vi "Forbidden.vi"() -> ()   [LabVIEW 2014]
panel:
  in  "menu":bool
  out "forbidden":bool[][](array[boolean])
  out "current col":dbl
  out "current row":dbl
  in  "redo":bool
  out "status":bool
  in  "resume":bool caption="restart"
  out "Game status":string
  out "?":bool
  out "?":bool
  out "counts":dbl
  out "white":bool[][](array[boolean])
  out "blackPiece":bool
  out "whitePiece":bool
  out "black":bool[][](array[boolean])
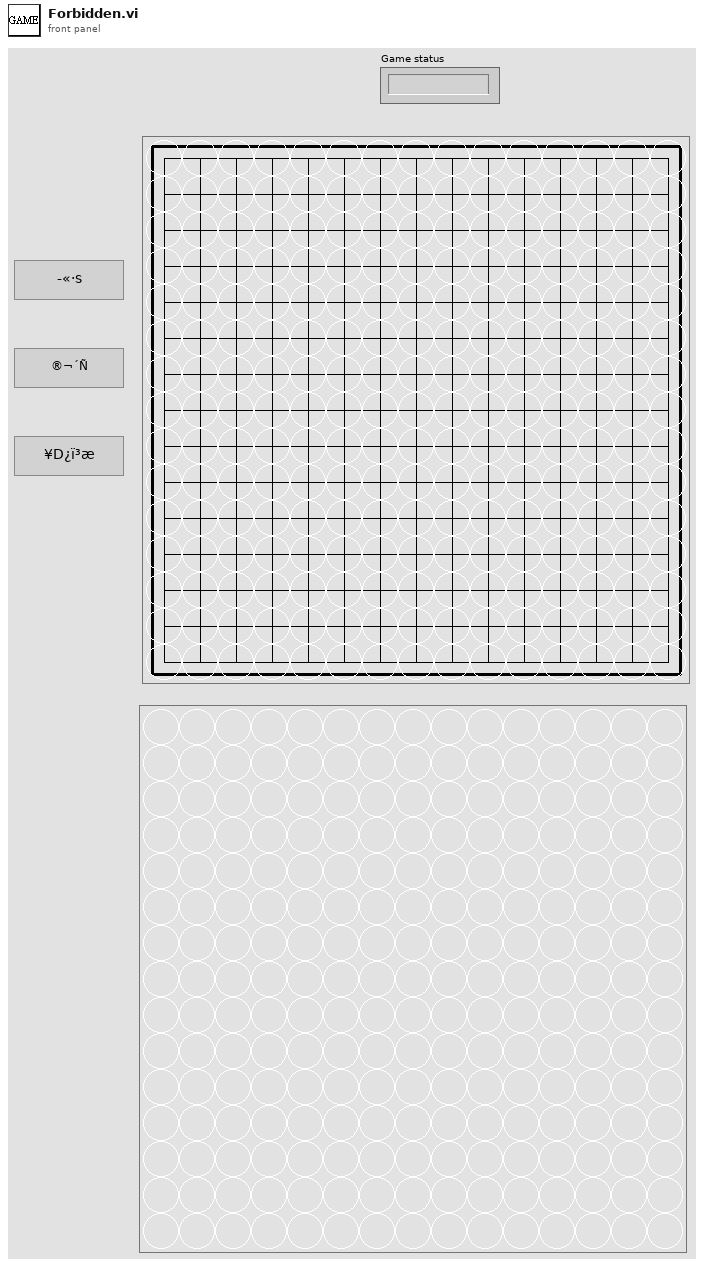
[diagram p1: front panel]
types:
  T1 = typedef "LVPoint32TypeDef.ctl" = cluster{"Horizontal":i32, "Vertical":i32}
  T2 = cluster{"Numeric Control":dbl, "Numeric Control":dbl}
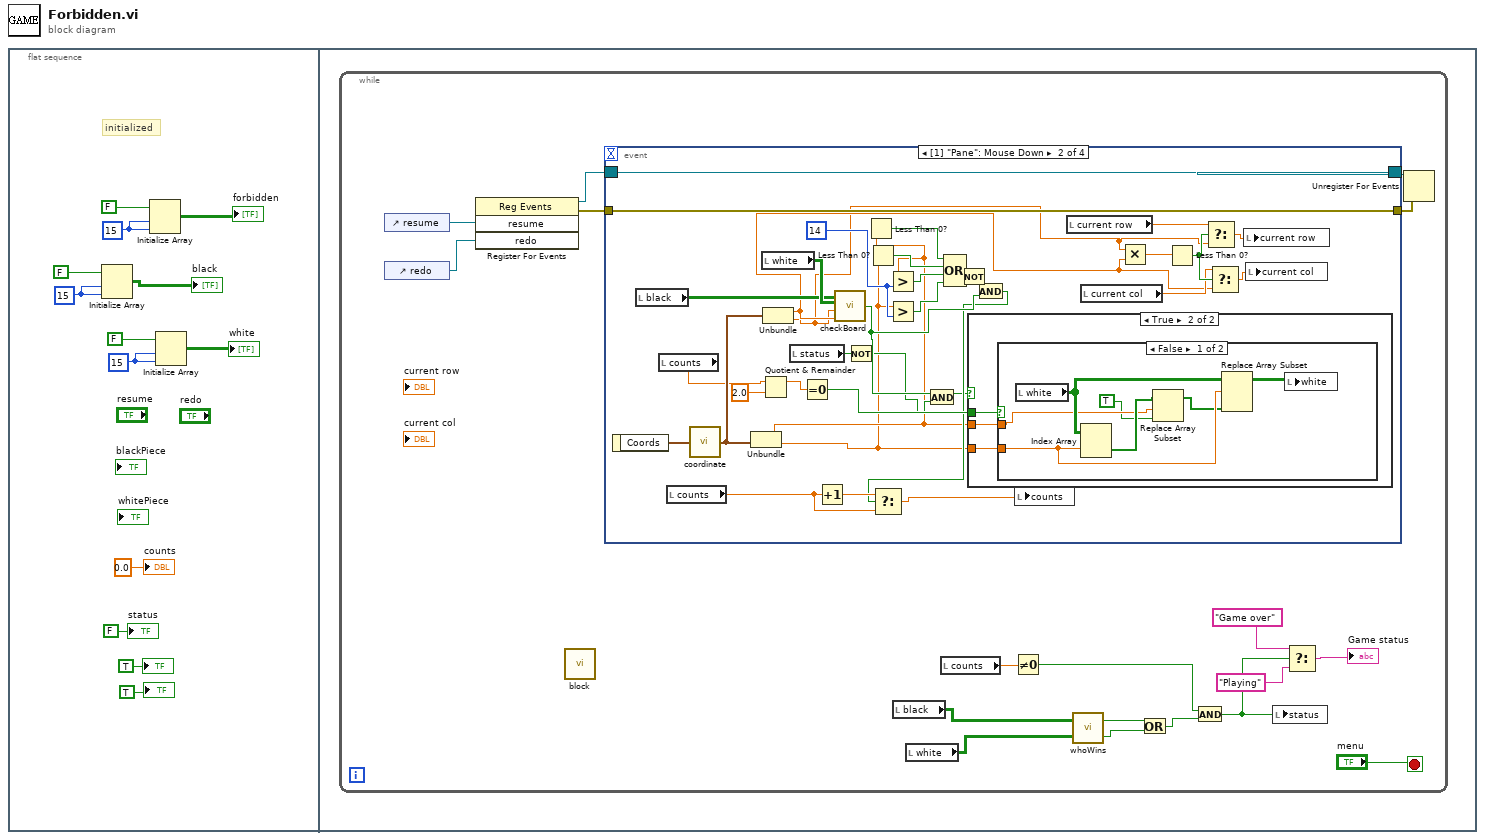
[diagram p0: block diagram]
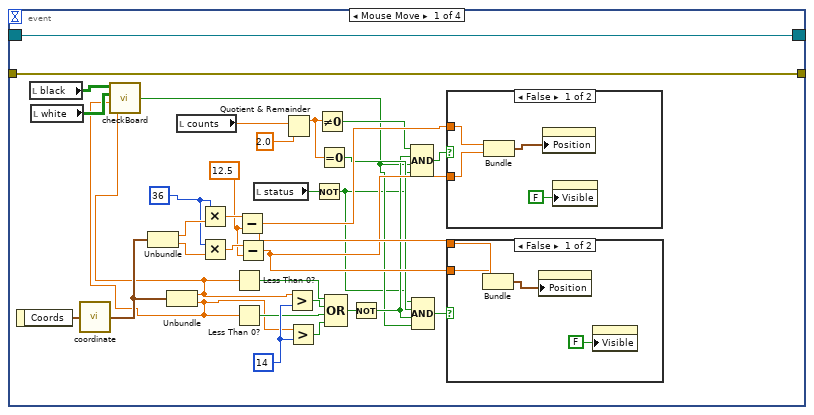
[diagram p2: hidden frame]
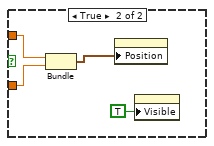
[diagram p3: hidden frame]
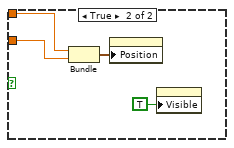
[diagram p4: hidden frame]
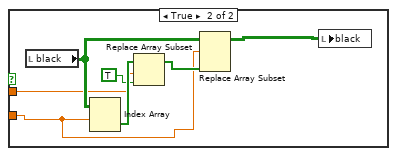
[diagram p6: hidden frame]
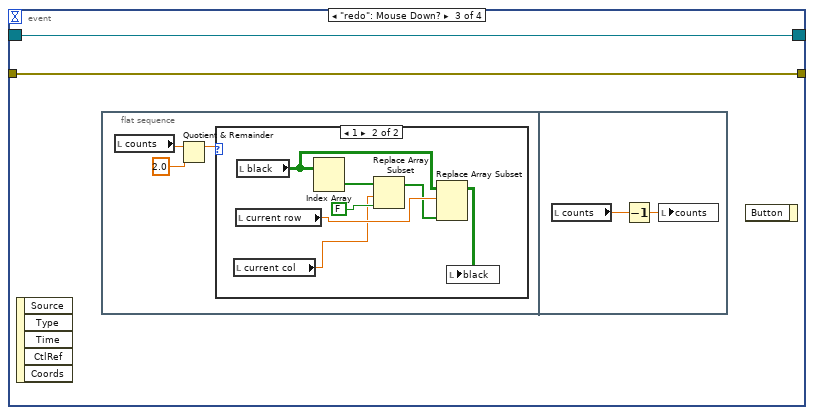
[diagram p7: hidden frame]
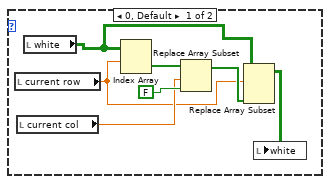
[diagram p8: hidden frame]
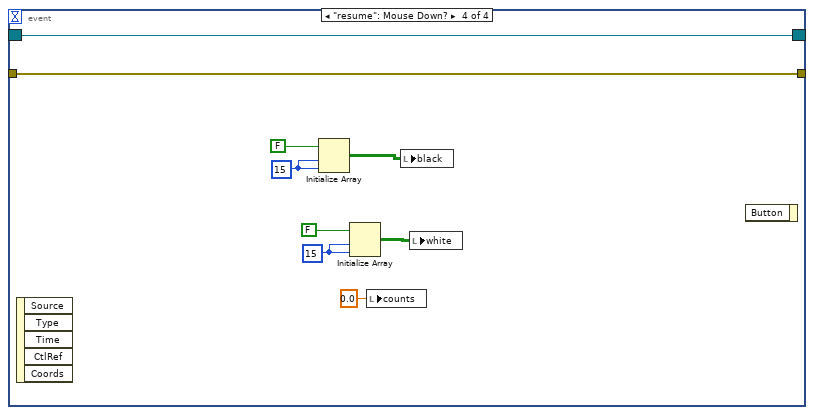
[diagram p9: hidden frame]
diagram:
  n1 = flat-sequence {
    frame #0 {
      w4 = 15
      w12 = 15
      w9 = 15
      # "initialized"
      n2 = Initialize Array(FALSE, w9, w9) -> (→"black":bool[][])
      n3 = Initialize Array(FALSE, w4, w4) -> (→"forbidden":bool[][])
      n4 = Initialize Array(FALSE, w12, w12) -> (→"white":bool[][])
      "counts" <- 0.0 ("Numeric Indicator")
      "status" <- FALSE ("status")
      "?" <- TRUE
      "?" <- TRUE
    }
    frame #1 {
      n5 = while {
        stop <- "menu" stop-if-true
        n6 = control-ref of="resume"() -> (w27:refnum<vi>)
        n7 = control-ref of="redo"() -> (w15:refnum<vi>)
        n8 = register-events(w27, w15) -> (reference out=w29:refnum<event-registration>, error out=w31:errorcluster)  [unwired: 2 in]
        n9 = call "block.vi"() -> ()  [unwired: 4 in, 1 out]
        n10 = event shown="[1] \"Pane\": Mouse Down" {
          selector: w29 -> [w64 w115 w134 w161]
          dyn-events: [w64 w115 w134 w161] -> w28
          timeout: _ -> [_ _ _ _]
          tunnel: w31 -> [w63 w114 w133 w160]
          tunnel: [w63 w114 w133 w160] -> w30
          event Mouse Move {
            w54 = 14
            w56 = 12.5
            w59 = 36
            n11 = event-data() -> ("Coords"=w62:T1)  [unwired: 1 in]
            n12 = local read "black"() -> (w38:bool[][])
            n13 = local read "white"() -> (w37:bool[][])
            n14 = call "coordinate.vi"("Cluster"=w62) -> ("output cluster"=w55:T2)
            n15 = Unbundle(w55) -> ("Numeric Control"=w61:dbl, "Numeric Control"=w60:dbl)
            n16 = Unbundle(w55) -> ("Numeric Control"=w36:dbl, "Numeric Control"=w35:dbl)
            n17 = call "checkBoard.vi"("column"=w36, "row"=w35, "white"=w37, "black"=w38) -> ("element"=w34:bool)
            n18 = local read "counts"() -> (w47:dbl)
            n19 = Multiply(x=w59, y=w61) -> (x*y=w58:dbl)
            n20 = Multiply(x=w59, y=w60) -> (x*y=w57:dbl)
            n21 = Less Than 0?(x=w36) -> (x < 0?=w53:bool)
            n22 = Less Than 0?(x=w35) -> (x < 0?=w51:bool)
            n23 = Subtract(x=w58, y=w56) -> (x-y=w49:dbl)
            n24 = Subtract(x=w57, y=w56) -> (x-y=w48:dbl)
            n25 = local read "status"() -> (w33:bool)
            n26 = Quotient & Remainder(x=w47, y=2.0) -> (x-y*floor(x/y)=w41:dbl)  [unwired: 1 out]
            n27 = Greater?(x=w36, y=w54) -> (0:w52:bool)
            n28 = Greater?(x=w35, y=w54) -> (0:w50:bool)
            n29 = Not(x=w33) -> (.not. x?=w32:bool)
            n30 = Not Equal To 0?(x=w41) -> (x != 0?=w42:bool)
            n31 = Equal To 0?(x=w41) -> (x = 0?=w40:bool)
            n32 = Compound Arithmetic op=OR(w53, w52, w51, w50) -> (w43:bool)
            n33 = Not(x=w43) -> (.not. x?=w39:bool)
            n34 = Compound Arithmetic op=AND(w42, w39, w34, w32) -> (w45:bool)
            n35 = Compound Arithmetic op=AND(w32, w40, w39, w34) -> (w44:bool)
            n36 = case shown="False" w45 {
              tunnel: w49 -> [w68 w71]
              tunnel: w48 -> [w67 w70]
              frame False {
                n37 = Bundle(w68, w67) -> (w66:cluster{dbl, dbl})  [unwired: 1 in]
                n38 = property class="Bool (strict)"("Position"=w66) -> ()  [unwired: 2 in, 2 out]
                n39 = property class="Bool (strict)"("Visible"=FALSE) -> ()  [unwired: 2 in, 2 out]
              }
              frame True {
                n40 = Bundle(w71, w70) -> (w69:cluster{dbl, dbl})  [unwired: 1 in]
                n41 = property class="Bool (strict)"("Position"=w69) -> ()  [unwired: 2 in, 2 out]
                n42 = property class="Bool (strict)"("Visible"=TRUE) -> ()  [unwired: 2 in, 2 out]
              }
            }
            n43 = case shown="False" w44 {
              tunnel: w49 -> [w75 w80]
              tunnel: w48 -> [w74 w79]
              frame False {
                n44 = Bundle(w75, w74) -> (w76:cluster{dbl, dbl})  [unwired: 1 in]
                n45 = property class="Bool (strict)"("Position"=w76) -> ()  [unwired: 2 in, 2 out]
                n46 = property class="Bool (strict)"("Visible"=FALSE) -> ()  [unwired: 2 in, 2 out]
              }
              frame True {
                n47 = Bundle(w80, w79) -> (w78:cluster{dbl, dbl})  [unwired: 1 in]
                n48 = property class="Bool (strict)"("Position"=w78) -> ()  [unwired: 2 in, 2 out]
                n49 = property class="Bool (strict)"("Visible"=TRUE) -> ()  [unwired: 2 in, 2 out]
              }
            }
          }
          event Mouse Down {
            w102 = 14
            n50 = event-data() -> ("Coords"=w113:T1)  [unwired: 1 in]
            n51 = local read "black"() -> (w107:bool[][])
            n52 = local read "counts"() -> (w111:dbl)
            n53 = local read "counts"() -> (w105:dbl)
            n54 = call "coordinate.vi"("Cluster"=w113) -> ("output cluster"=w112:T2)
            n55 = Unbundle(w112) -> ("Numeric Control"=w90:dbl, "Numeric Control"=w89:dbl)
            n56 = Quotient & Remainder(x=w111, y=2.0) -> (x-y*floor(x/y)=w109:dbl)  [unwired: 1 out]
            n57 = local read "white"() -> (w108:bool[][])
            n58 = Unbundle(w112) -> ("Numeric Control"=w83:dbl, "Numeric Control"=w82:dbl)
            n59 = local read "status"() -> (w92:bool)
            n60 = Equal To 0?(x=w109) -> (x = 0?=w106:bool)
            n61 = Increment(x=w105) -> (x+1=w103:dbl)
            n62 = call "checkBoard.vi"("column"=w83, "row"=w82, "white"=w108, "black"=w107) -> ("element"=w96:bool)
            n63 = Not(x=w92) -> (.not. x?=w91:bool)
            n64 = Less Than 0?(x=w90) -> (x < 0?=w101:bool)
            n65 = Less Than 0?(x=w89) -> (x < 0?=w100:bool)
            n66 = Greater?(x=w90, y=w102) -> (0:w99:bool)
            n67 = Greater?(x=w89, y=w102) -> (0:w98:bool)
            n68 = And(x=w96, y=w91) -> (x .and. y?=w93:bool)
            n69 = Compound Arithmetic op=OR(w101, w100, w99, w98) -> (w97:bool)
            n70 = Not(x=w97) -> (.not. x?=w94:bool)
            n71 = case shown="True" w93 {
              tunnel: w90 -> [_ w118]
              tunnel: w89 -> [_ w117]
              tunnel: w106 -> [_ w116]
              frame False {
              }
              frame True {
                n72 = case shown="False" w116 {
                  tunnel: w118 -> [w121 w127]
                  tunnel: w117 -> [w123 w126]
                  frame False {
                    n73 = local read "white"() -> (w125:bool[][])
                    n74 = Index Array(array=w125, index (row)=w123) -> (element=w122:bool[])  [unwired: 1 in]
                    n75 = Replace Array Subset(array=w122, new element=TRUE, index=w121) -> (w119:bool[])
                    n76 = Replace Array Subset(array=w125, new element=w119, index (row)=w123) -> (w124:bool[][])  [unwired: 1 in]
                    n77 = local write "white"(w124) -> ()
                  }
                  frame True {
                    n78 = local read "black"() -> (w129:bool[][])
                    n79 = Index Array(array=w129, index (row)=w126) -> (element=w132:bool[])  [unwired: 1 in]
                    n80 = Replace Array Subset(array=w132, new element=TRUE, index=w127) -> (w130:bool[])
                    n81 = Replace Array Subset(array=w129, new element=w130, index (row)=w126) -> (w128:bool[][])  [unwired: 1 in]
                    n82 = local write "black"(w128) -> ()
                  }
                }
              }
            }
            n83 = And(x=w94, y=w96) -> (x .and. y?=w95:bool)
            n84 = Select(t=w103, s=w95, f=w105) -> (s? t:f=w104:dbl)
            n85 = local write "counts"(w104) -> ()
            n86 = local read "current row"() -> (w87:dbl)
            n87 = local read "current col"() -> (w84:dbl)
            n88 = Multiply(x=w82, y=w83) -> (x*y=w88:dbl)
            n89 = Less Than 0?(x=w88) -> (x < 0?=w85:bool)
            n90 = Select(t=w87, s=w85, f=w82) -> (s? t:f=w86:dbl)
            n91 = Select(t=w84, s=w85, f=w83) -> (s? t:f=w81:dbl)
            n92 = local write "current row"(w86) -> ()
            n93 = local write "current col"(w81) -> ()
          }
          event "redo": Mouse Down? {
            n94 = event-data() -> ()  [unwired: 1 in, 5 out]
            n95 = flat-sequence {
              frame #0 {
                n96 = local read "counts"() -> (w137:dbl)
                n97 = Quotient & Remainder(x=w137, y=2.0) -> (x-y*floor(x/y)=w135:dbl)  [unwired: 1 out]
                n98 = case shown="1" w135 {
                  frame 0, Default {
                    n99 = local read "current row"() -> (w140:dbl)
                    n100 = local read "current col"() -> (w142:dbl)
                    n101 = local read "white"() -> (w139:bool[][])
                    n102 = Index Array(array=w139, index (row)=w140) -> (element=w144:bool[])  [unwired: 1 in]
                    n103 = Replace Array Subset(array=w144, new element=FALSE, index=w142) -> (w141:bool[])
                    n104 = Replace Array Subset(array=w139, new element=w141, index (row)=w140) -> (w138:bool[][])  [unwired: 1 in]
                    n105 = local write "white"(w138) -> ()
                  }
                  frame 1 {
                    n106 = local read "current col"() -> (w148:dbl)
                    n107 = local read "current row"() -> (w149:dbl)
                    n108 = local read "black"() -> (w147:bool[][])
                    n109 = Index Array(array=w147) -> (element=w151:bool[])  [unwired: 2 in]
                    n110 = Replace Array Subset(array=w151, new element=FALSE, index=w148) -> (w145:bool[])
                    n111 = Replace Array Subset(array=w147, new element=w145, index (row)=w149) -> (w146:bool[][])  [unwired: 1 in]
                    n112 = local write "black"(w146) -> ()
                  }
                }
              }
              frame #1 {
                n113 = local read "counts"() -> (w153:dbl)
                n114 = Decrement(x=w153) -> (x-1=w152:dbl)
                n115 = local write "counts"(w152) -> ()
              }
            }
            n116 = event-data() -> ()  [unwired: 2 in, 1 out]
          }
          event "resume": Mouse Down? {
            w156 = 15
            w159 = 15
            n117 = event-data() -> ()  [unwired: 1 in, 5 out]
            n118 = Initialize Array(FALSE, w156, w156) -> (w154:bool[][])
            n119 = Initialize Array(FALSE, w159, w159) -> (w157:bool[][])
            n120 = local write "counts"(0.0 ("counts")) -> ()
            n121 = local write "black"(w154) -> ()
            n122 = local write "white"(w157) -> ()
            n123 = event-data() -> ()  [unwired: 2 in, 1 out]
          }
        }
        n124 = local read "black"() -> (w17:bool[][])
        n125 = local read "white"() -> (w18:bool[][])
        n126 = local read "counts"() -> (w21:dbl)
        n127 = Not Equal To 0?(x=w21) -> (x != 0?=w22:bool)
        n128 = call "whoWins.vi"("white"=w18, "black"=w17) -> ("wWins"=w20:bool, "bWins"=w19:bool)
        n129 = Or(x=w19, y=w20) -> (x .or. y?=w23:bool)
        n130 = And(x=w22, y=w23) -> (x .and. y?=w16:bool)
        n131 = local write "status"(w16) -> ()
        n132 = Select(t="Game over", s=w16, f="Playing") -> (s? t:f=→"Game status":string)
        n133 = Unregister For Events(event registration refnum=w28, error in=w30) -> ()  [unwired: 1 out]
      }
    }
  }
